vi "Recursive VI Search.vi"(8 "error in (no error)":errorcluster, 10 "Project Item":refnum<vi>) -> (0 "error out":errorcluster, 2 "VI Paths":path[](array[path]))   [LabVIEW 2018]
doc: "This VI does a recersive look in project items to look for VIs."
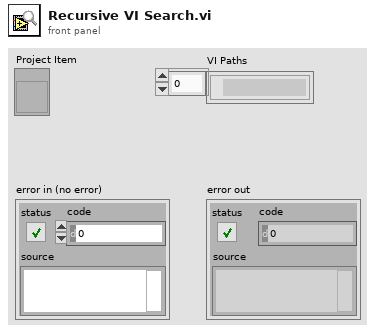
[diagram p1: front panel]
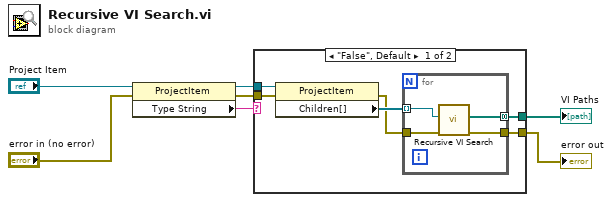
[diagram p0: block diagram]
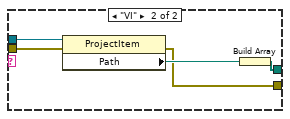
[diagram p2: hidden frame]
diagram:
  n1 = property class="ProjectItem"(reference="Project Item", error in="error in (no error)") -> (reference out=w5:refnum<vi>, error out=w4:errorcluster, "Type String"=w6:string)
  n2 = case shown="\"False\", Default" w6 {
    tunnel: w5 -> [w13 w22]
    tunnel: w4 -> [w9 w21]
    tunnel: [w8 w19] -> w3
    tunnel: [w10 w18] -> w1
    frame "False", Default {
      n3 = property class="ProjectItem"(reference=w13, error in=w9) -> (error out=w11:errorcluster, "Children[]"=w12:refnum<vi>[])  [unwired: 1 out]
      n4 = for {
        tunnel: w12 -> [w14] mode=indexing
        tunnel: w11 -> [w17]
        tunnel: [w16] -> w10
        tunnel: [w15] -> w8 mode=concatenating
        n5 = call "Recursive VI Search.vi"("error in (no error)"=w17, "Project Item"=w14) -> ("error out"=w16:errorcluster, "VI Paths"=w15:path[])  [unwired: 8 in]
      }
    }
    frame "VI" {
      n6 = property class="ProjectItem"(reference=w22, error in=w21) -> (error out=w18:errorcluster, "Path"=w20:path)  [unwired: 1 out]
      n7 = Build Array(w20) -> (w19:path[])
    }
  }
  "VI Paths" <- w3
  "error out" <- w1
